vi "F020_time32_set.vi"(8 "error in":errorcluster, 10 "Cluster":cluster{"ADDRESS":u8, "time_U32":u32}={"ADDRESS"=170, "time_U32"=170} {"time_U32" format="%.0x"; "ADDRESS" format="%.0x"}, 11 "COM in":string="COM4") -> (0 "error out":errorcluster={"status"=TRUE, "code"=-1073807343, "source"=""}, 2 "TIME32":u32 format="%.0x", 3 "COM out":string="COM4")   [LabVIEW 2016]
doc: "This example performs a serial port write and a serial port read. The parameters set for the serial port must match the parameters of the connected instrument or device. The VISA Configure Serial Port VI sets the configuration parameters. The front panel displays the controls used to configure the basic parameters, such as baud rate, data bits, and parity. The VI passes the VISA resource name to other VIs that perform operations on that VISA resource. The VISA Write function sends a command to the serial device and the VISA Read function returns data based on the command. The VISA Close function then closes the reference to the serial device. It is important to close the reference; otherwise, further communication through that port might not be possible."
panel:
  # "loopback: <xxAABB>\nwr_dout:   <xxAA11aabbccdd> aa=ch, bb=val, ccdd=timeout[sec]\nrd_ain:      <xxAA13aa> -> {qqww}"
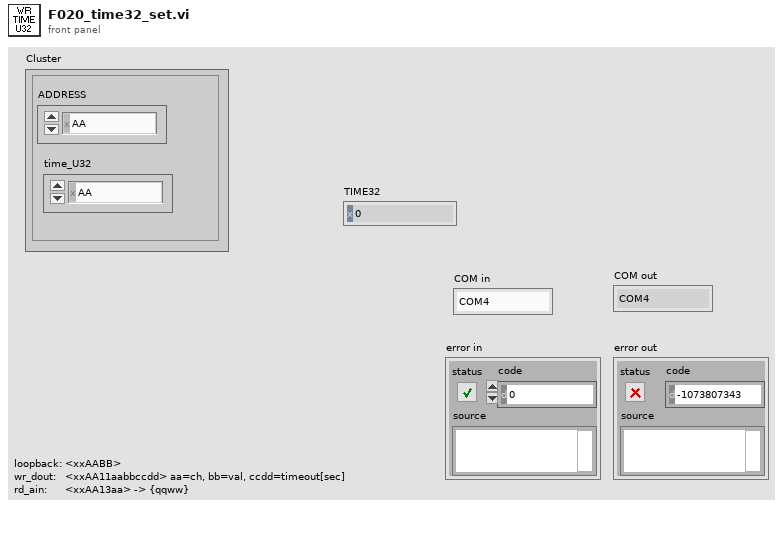
[diagram p1: front panel]
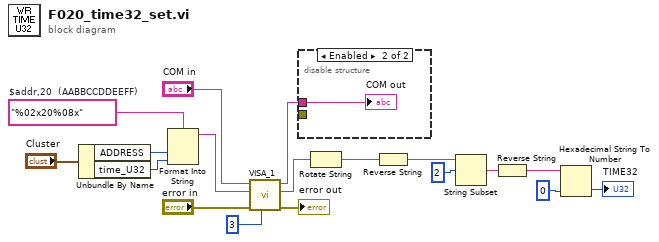
[diagram p0: block diagram]
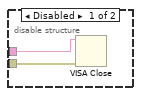
[diagram p2: hidden frame]
diagram:
  w15 = "%02x20%08x"  # $addr,20  (AABBCCDDEEFF)
  n1 = Unbundle By Name("Cluster") -> ("ADDRESS"=w12:u8, "time_U32"=w13:u32)
  n2 = Format Into String(format string=w15, w12, w13) -> (resulting string=w10:string)  [unwired: 2 in, 1 out]
  n3 = call "VISA_1.vi"("delay[ms]"=u32 3, "error in"="error in", "wr_buf"=w10, "COM in"="COM in") -> ("error out"=→"error out":errorcluster, "rx_buf"=w11:string, "COM out"=w18:string)  [unwired: 4 in, 1 out]
  n4 = disable-structure shown="Enabled" {
    disable-tunnel: _ -> [w20 _]
    disable-tunnel: w18 -> [w19 w21]
    frame Disabled {
      n5 = VISA Close(VISA resource name=w19, error in (no error)=w20) -> ()  [unwired: 1 out]
    }
    frame Enabled {
      "COM out" <- w21
    }
  }
  n6 = Rotate String(1:w11) -> (0:w3:string)
  n7 = Reverse String(1:w3) -> (0:w4:string)
  n8 = String Subset(string=w4, offset (0)=2) -> (substring=w6:string)  [unwired: 1 in]
  n9 = Reverse String(1:w6) -> (0:w8:string)
  n10 = Hexadecimal String To Number(string=w8, default (0uL)=u32 0 ("default (0 U32)")) -> (number=→"TIME32":u32)  [unwired: 1 in, 1 out]
